vi "Test - Calculate Display Position.vi"   [LabVIEW 2018, in "Camera.lvclass"]
uses:
  Camera.lvclass
  <vilib>/addons/_JKI Toolkits/Caraya/classes/Test/Test.lvclass
  LabSDL2/Source/Libraries/SDL2 Utility/Point (I32).ctl
  LabSDL2/Source/Libraries/SDL2 Utility/SDL2 Utility.lvlib
  <vilib>/addons/_JKI Toolkits/Caraya/classes/Assert/Assert.lvclass
types:
  T1 = typedef "SDL2 Utility.lvlib/Point (I32).ctl" = cluster{"x":i32, "y":i32}
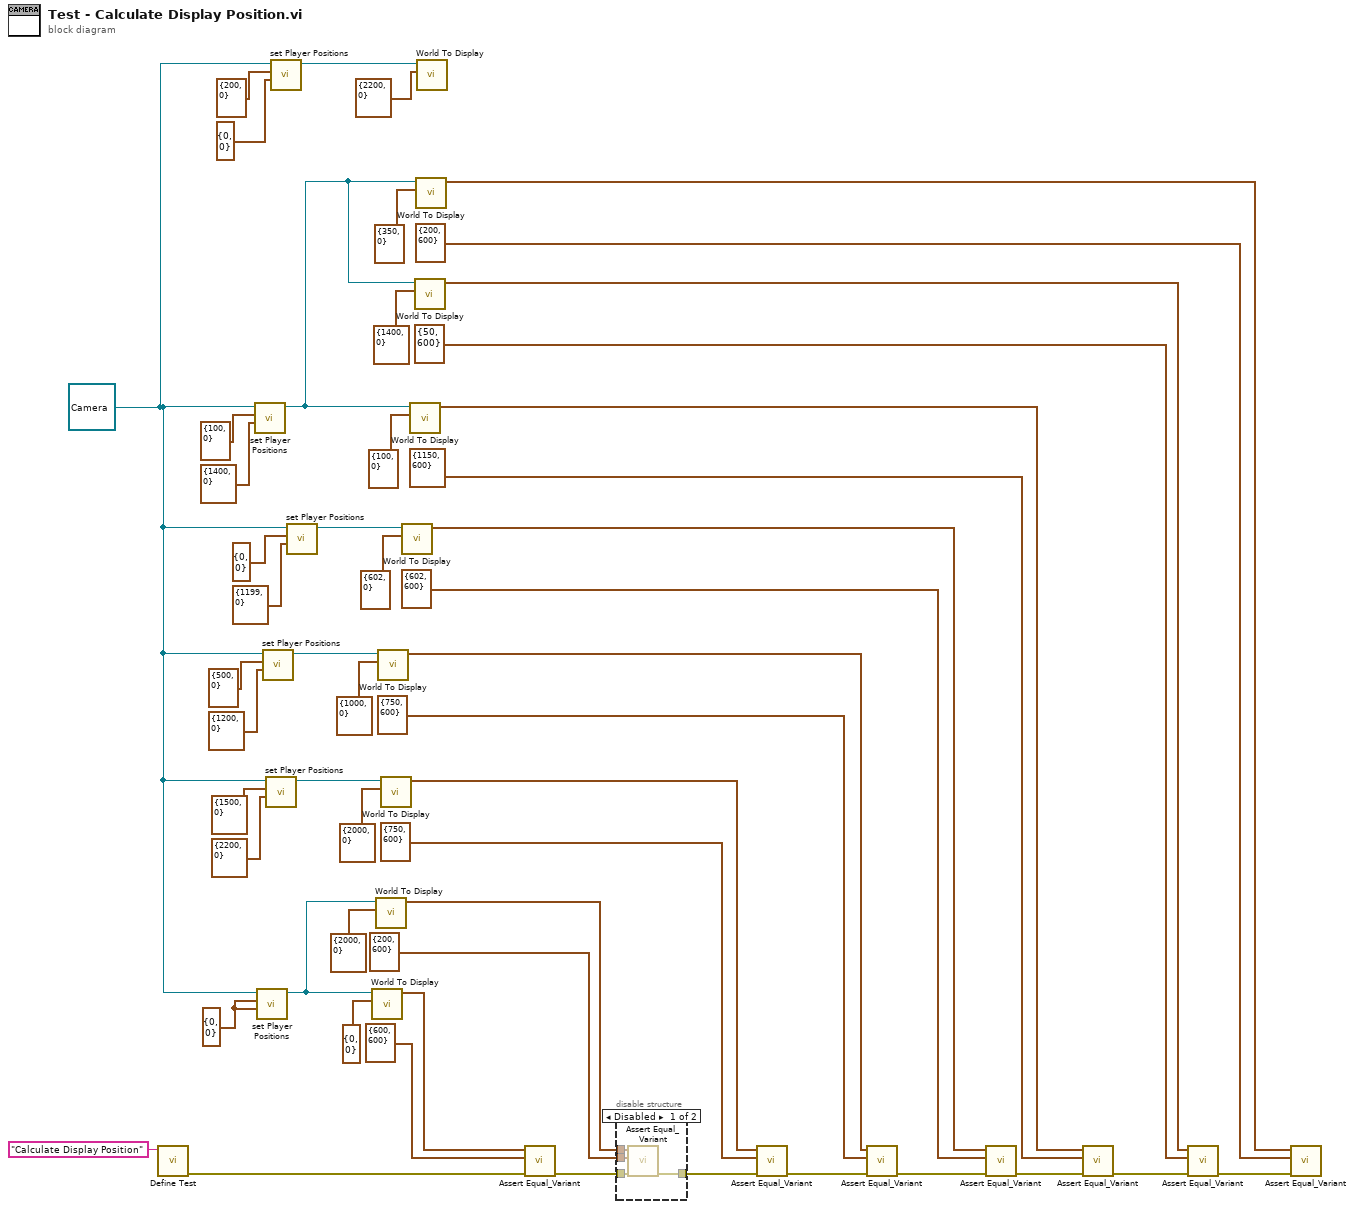
[diagram p0: block diagram]
diagram:
  w17 = T1 {"x"=0, "y"=0} ("Player 1 World Position")
  w3 = refnum<class "Camera.lvclass"> refnum ("Camera.lvclass")
  n1 = call <vilib>:"Define Test.vi"("Label (VI Title)"="Calculate Display Position") -> ("error out"=w50:errorcluster)  [unwired: 10 in]
  n2 = call "set Player Positions.vi"("Player 2 Position"=T1 {"x"=1400, "y"=0} ("Player 1 World Position"), "Player 1 Position"=T1 {"x"=100, "y"=0} ("Player 1 World Position"), "Camera in"=w3) -> ("Camera out"=w28:refnum<class "Camera.lvclass">)  [unwired: 8 in]
  n3 = call "set Player Positions.vi"("Player 2 Position"=w17, "Player 1 Position"=w17, "Camera in"=w3) -> ("Camera out"=w10:refnum<class "Camera.lvclass">)  [unwired: 8 in]
  n4 = call "set Player Positions.vi"("Player 2 Position"=T1 {"x"=1200, "y"=0} ("Player 1 World Position"), "Player 1 Position"=T1 {"x"=500, "y"=0} ("Player 1 World Position"), "Camera in"=w3) -> ("Camera out"=w13:refnum<class "Camera.lvclass">)  [unwired: 8 in]
  n5 = call "set Player Positions.vi"("Player 2 Position"=T1 {"x"=2200, "y"=0} ("Player 1 World Position"), "Player 1 Position"=T1 {"x"=1500, "y"=0} ("Player 1 World Position"), "Camera in"=w3) -> ("Camera out"=w20:refnum<class "Camera.lvclass">)  [unwired: 8 in]
  n6 = call "set Player Positions.vi"("Player 2 Position"=T1 {"x"=0, "y"=0} ("Player 1 World Position"), "Player 1 Position"=T1 {"x"=200, "y"=0} ("Player 1 World Position"), "Camera in"=w3) -> ("Camera out"=w2:refnum<class "Camera.lvclass">)  [unwired: 8 in]
  n7 = call "set Player Positions.vi"("Player 2 Position"=T1 {"x"=1199, "y"=0} ("Player 1 World Position"), "Player 1 Position"=T1 {"x"=0, "y"=0} ("Player 1 World Position"), "Camera in"=w3) -> ("Camera out"=w24:refnum<class "Camera.lvclass">)  [unwired: 8 in]
  n8 = call "World To Display.vi"("World Position"=T1 {"x"=0, "y"=0} ("Player 1 World Position"), "Camera in"=w10) -> ("Display Position"=w49:T1)  [unwired: 9 in]
  n9 = call "World To Display.vi"("World Position"=T1 {"x"=2000, "y"=0} ("Player 1 World Position"), "Camera in"=w10) -> ("Display Position"=w8:T1)  [unwired: 9 in]
  n10 = call "World To Display.vi"("World Position"=T1 {"x"=1000, "y"=0} ("Player 1 World Position"), "Camera in"=w13) -> ("Display Position"=w45:T1)  [unwired: 9 in]
  n11 = call "World To Display.vi"("World Position"=T1 {"x"=2000, "y"=0} ("Player 1 World Position"), "Camera in"=w20) -> ("Display Position"=w48:T1)  [unwired: 9 in]
  n12 = call "World To Display.vi"("World Position"=T1 {"x"=602, "y"=0} ("Player 1 World Position"), "Camera in"=w24) -> ("Display Position"=w42:T1)  [unwired: 9 in]
  n13 = call "World To Display.vi"("World Position"=T1 {"x"=100, "y"=0} ("Player 1 World Position"), "Camera in"=w28) -> ("Display Position"=w39:T1)  [unwired: 9 in]
  n14 = call "World To Display.vi"("World Position"=T1 {"x"=1400, "y"=0} ("Player 1 World Position"), "Camera in"=w28) -> ("Display Position"=w36:T1)  [unwired: 9 in]
  n15 = call "World To Display.vi"("World Position"=T1 {"x"=350, "y"=0} ("Player 1 World Position"), "Camera in"=w28) -> ("Display Position"=w32:T1)  [unwired: 9 in]
  n16 = call "World To Display.vi"("World Position"=T1 {"x"=2200, "y"=0} ("Player 1 World Position"), "Camera in"=w2) -> ()  [unwired: 9 in, 1 out]
  n17 = call <vilib>:"Assert Equal_Variant.vi"("error in (no error)"=w50, "Y"=T1 {"x"=600, "y"=600} ("Player 1 World Position"), "X"=w49) -> ("error out"=w9:errorcluster)  [unwired: 8 in]
  n18 = disable-structure shown="Disabled" {
    disable-tunnel: w9 -> [w56 w57]
    disable-tunnel: w8 -> [w55 _]
    disable-tunnel: T1 {"x"=200, "y"=600} ("Player 1 World Position") -> [w54 _]
    disable-tunnel: [w53 w57] -> w6
    frame Disabled {
      n19 = call <vilib>:"Assert Equal_Variant.vi"("error in (no error)"=w56, "Y"=w54, "X"=w55) -> ("error out"=w53:errorcluster)  [unwired: 8 in]
    }
    frame Enabled {
    }
  }
  n20 = call <vilib>:"Assert Equal_Variant.vi"("error in (no error)"=w6, "Y"=T1 {"x"=750, "y"=600} ("Player 1 World Position"), "X"=w48) -> ("error out"=w46:errorcluster)  [unwired: 8 in]
  n21 = call <vilib>:"Assert Equal_Variant.vi"("error in (no error)"=w46, "Y"=T1 {"x"=750, "y"=600} ("Player 1 World Position"), "X"=w45) -> ("error out"=w43:errorcluster)  [unwired: 8 in]
  n22 = call <vilib>:"Assert Equal_Variant.vi"("error in (no error)"=w43, "Y"=T1 {"x"=602, "y"=600} ("Player 1 World Position"), "X"=w42) -> ("error out"=w40:errorcluster)  [unwired: 8 in]
  n23 = call <vilib>:"Assert Equal_Variant.vi"("error in (no error)"=w40, "Y"=T1 {"x"=1150, "y"=600} ("Player 1 World Position"), "X"=w39) -> ("error out"=w37:errorcluster)  [unwired: 8 in]
  n24 = call <vilib>:"Assert Equal_Variant.vi"("error in (no error)"=w37, "Y"=T1 {"x"=50, "y"=600} ("Player 1 World Position"), "X"=w36) -> ("error out"=w33:errorcluster)  [unwired: 8 in]
  n25 = call <vilib>:"Assert Equal_Variant.vi"("error in (no error)"=w33, "Y"=T1 {"x"=200, "y"=600} ("Player 1 World Position"), "X"=w32) -> ()  [unwired: 8 in, 1 out]
